vi "View File.vi"(8 "error in":errorcluster, 11 "TDMS in":refnum<class "TDMS.lvclass">) -> (0 "error out":errorcluster, 3 "TDMS out":refnum<class "TDMS.lvclass">)   [LabVIEW 2020, in "Manejador archivo.lvlib" / "TDMS.lvclass"]
uses:
  TDMS.lvclass
  C:/GitClones/DQMH-LabVIEW-GYM/10 Mayo/04 DQMH USER/Libraries/Manejador archivo/Class Definitions/File/File.lvclass
  File/File.lvclass/File.ctl
  File/Read File Path.vi
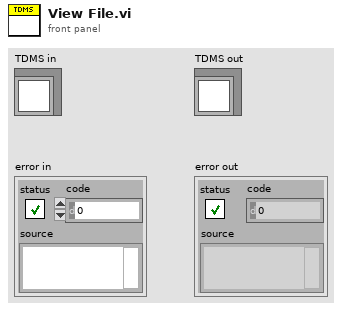
[diagram p1: front panel]
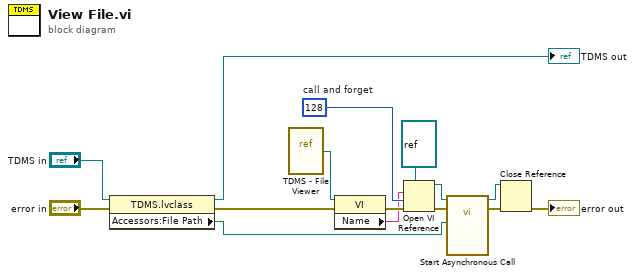
[diagram p0: block diagram]
diagram:
  w7 = 128  # call and forget
  n1 = property class="TDMS.lvclass"(reference="TDMS in", error in="error in") -> (reference out=→"TDMS out":refnum<class "TDMS.lvclass">, error out=w10:errorcluster, "Accessors:File Path"=w1:path)
  n2 = vi-ref <vilib>:"TDMS - File Viewer.vi"() -> (w4:refnum<vi>)
  n3 = property class="VI"(reference=w4, error in=w10) -> (error out=w14:errorcluster, "Name"=w5:string)  [unwired: 1 out]
  n4 = Open VI Reference(type specifier VI Refnum (for type only)=refnum<vi> refnum, vi path=w5, options=w7, error in (no error)=w14) -> (vi reference=w2:refnum<vi>, error out=w13:errorcluster)  [unwired: 2 in]
  n5 = call-by-ref "Start Asynchronous Call"(reference=w2, error in=w13, "file path"=w1) -> (reference out=w6:refnum<vi>, error out=w12:errorcluster)  [unwired: 5 in, 2 out]
  n6 = Close Reference(reference=w6, error in (no error)=w12) -> (error out=→"error out":errorcluster)
